vi "integracao.vi"() -> ()   [LabVIEW 2011]
panel:
  out "tempo":dbl
  out "Boolean 2":bool
  out "Waveform Chart 2":dynamicdata(graph)
  out "Boolean":bool
  out "slop curve":dbl
  out "Result":dbl
  out "Waveform Chart":dynamicdata(graph)
  in  "Filename":path=path "C:/works/CG3000/datalog/gc3000_15-03-31_1222.lvm"
  out "signal":dbl
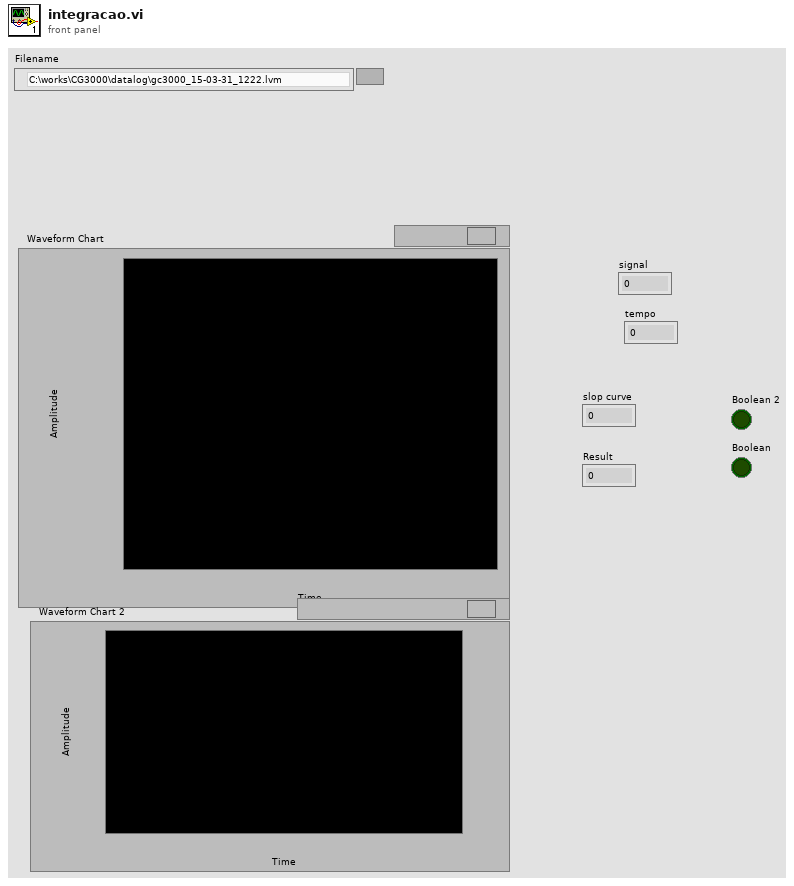
[diagram p1: front panel]
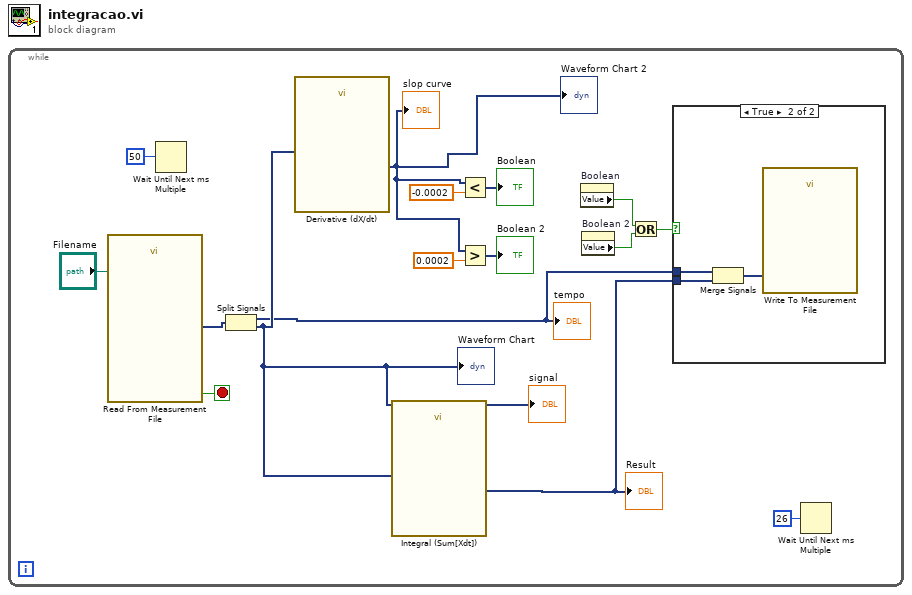
[diagram p0: block diagram]
diagram:
  n1 = while {
    stop <- w15 stop-if-true
    n2 = call "Read From Measurement File"("Filename"="Filename") -> ("Signals"=w8:dynamicdata, "EOF?"=w15:bool)  [unwired: 5 in, 4 out]
    n3 = Wait Until Next ms Multiple(millisecond multiple=u32 50) -> ()  [unwired: 1 out]
    n4 = Split Signals(w8) -> (w6:dynamicdata, w7:dynamicdata)  [unwired: 2 in]
    "signal" <- w7
    "Waveform Chart" <- w7
    "tempo" <- w6
    n5 = call "Derivative (dX/dt)"("Signals"=w7) -> ("Result"=w11:dynamicdata)  [unwired: 5 in, 1 out]
    "slop curve" <- w11
    "Waveform Chart 2" <- w11
    n6 = call "Integral (Sum[Xdt])"("Signals"=w7) -> ("Result"=w5:dynamicdata)  [unwired: 5 in, 1 out]
    "Result" <- w5
    n7 = Less?(x=w11, y=-0.0002) -> (x < y?=→"Boolean":dynamicdata)
    n8 = Greater?(x=w11, y=0.0002) -> (0:→"Boolean 2":dynamicdata)
    n9 = property on="Boolean" class="Bool (strict)"() -> ("Value"=w3:bool)  [unwired: 2 in, 2 out]
    n10 = property on="Boolean 2" class="Bool (strict)"() -> ("Value"=w2:bool)  [unwired: 2 in, 2 out]
    n11 = Or(x=w3, y=w2) -> (x .or. y?=w1:bool)
    n12 = case shown="True" w1 {
      tunnel: w6 -> [_ w18]
      tunnel: w5 -> [_ w17]
      frame False {
      }
      frame True {
        n13 = Merge Signals(w18, w17) -> (w19:dynamicdata)
        n14 = call "Write To Measurement File"("Signals"=w19) -> ()  [unwired: 16 in, 3 out]
      }
    }
    n15 = Wait Until Next ms Multiple(millisecond multiple=u32 26) -> ()  [unwired: 1 out]
  }
